vi "Logitech F310 (No Drivers).vi"(6 "error in (no error)":errorcluster, 7 "Deadzone":dbl=0.05, 8 "refnum name":string) -> (0 "Buttons":T2, 1 "D-Pad Buttons":T1, 2 "D-Pad":cluster{"X":dbl, "Y":dbl}, 3 "Right Stick":cluster{"X":dbl, "Y":dbl}, 4 "error out":errorcluster, 5 "Left Stick":cluster{"X":dbl, "Y":dbl})   [LabVIEW 2012]
uses:
  <vilib>/Rock Robotics/WPI/Joystick/WPI_JoystickGetSetRefNum.vi
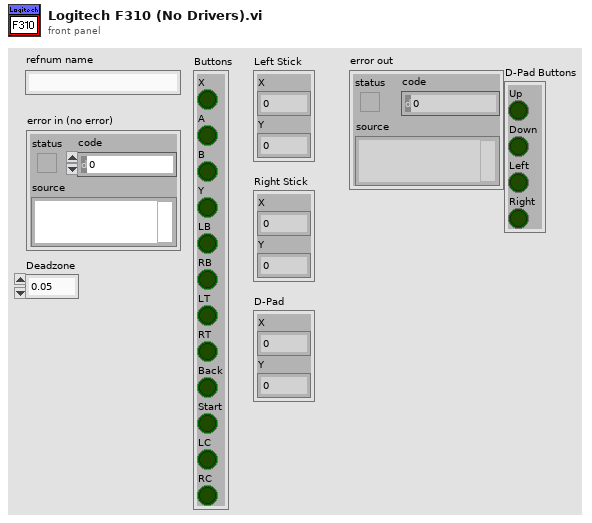
[diagram p1: front panel]
types:
  T1 = cluster{"Up":bool, "Down":bool, "Left":bool, "Right":bool}
  T2 = cluster{"X":bool, "A":bool, "B":bool, "Y":bool, "LB":bool, "RB":bool, "LT":bool, "RT":bool, "Back":bool, "Start":bool, "LC":bool, "RC":bool}
  T3 = typedef "WPI_JoystickDevRef.ctl" = cluster{"Device":T4}
  T4 = typedef "WPI_JoystickDeviceEnum.ctl" = enum16{"USB 1", "USB 2", "USB 3", "USB 4", "Kinect 1", "Kinect 2"}
  T5 = typedef "WPI_JoystickButtonState.ctl" = cluster{"Button 1":bool, "Button 2":bool, "Button 3":bool, "Button 4":bool, "Button 5":bool, "Button 6":bool, "Button 7":bool, "Button 8":bool, "Button 9":bool, "Button 10":bool, "Button 11":bool, "Button 12":bool}
  T6 = cluster{"axis 1 (x)":dbl, "axis 2 (y)":dbl, "axis 3 (throttle)":dbl, "axis 4":dbl, "axis 5":dbl, "axis 6":dbl}
  T7 = cluster{"Array(out)[0]":dbl, "Array(out)[1]":dbl, "Array(out)[2]":dbl, "Array(out)[3]":dbl, "Array(out)[4]":dbl, "Array(out)[5]":dbl}
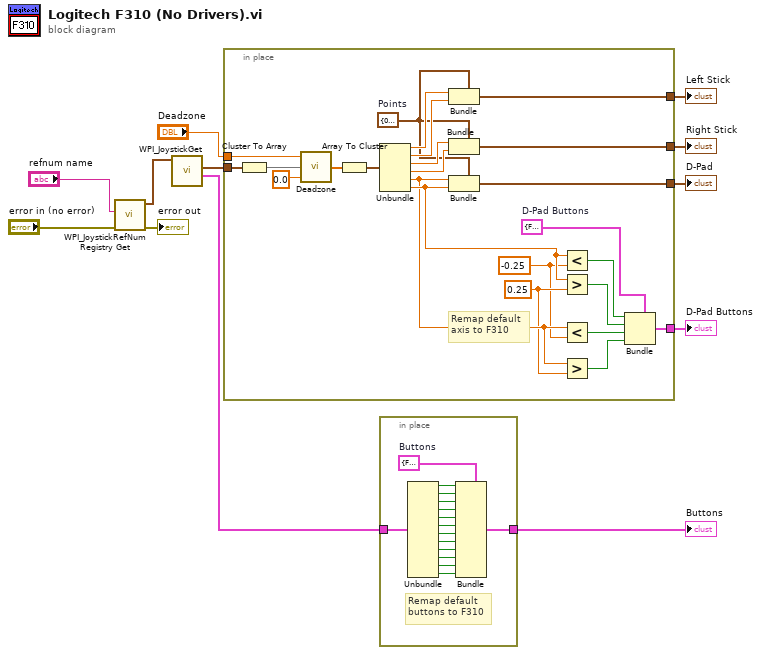
[diagram p0: block diagram]
diagram:
  n1 = call <vilib>:"WPI_JoystickRefNum Registry Get.vi"("error in (no error)"="error in (no error)", "refnum name"="refnum name") -> ("error out"=→"error out":errorcluster, "JoystickDevRef"=w12:T3)  [unwired: 8 in]
  n2 = call <vilib>:"WPI_JoystickGet.vi"("JoystickDevRef"=w12) -> ("Buttons"=w10:T5, "Axes"=w11:T6)  [unwired: 4 in, 1 out]
  n3 = in-place {
    in-place-border: w11 -> [w16]
    in-place-border: [w32] -> w6
    in-place-border: [w31] -> w5
    in-place-border: [w29] -> w4
    in-place-border: [w23] -> w2
    in-place-border: "Deadzone" -> [w13]
    w24 = -0.25 ("y")
    w25 = 0.25 ("y")
    w28 = T1 {"Up"=FALSE, "Down"=FALSE, "Left"=FALSE, "Right"=FALSE}  # D-Pad Buttons
    w30 = cluster{"X":dbl, "Y":dbl} {"X"=0.0, "Y"=0.0}  # Points
    # "Remap default\naxis to F310"
    n4 = Cluster To Array(cluster=w16) -> (array=w18:dbl[])
    n5 = call "Deadzone.vi"("Default"=0.0, "Array(in)"=w18, "Deadzone"=w13) -> ("Array(out)"=w17:dbl[])  [unwired: 2 in]
    n6 = Array To Cluster(array=w17) -> (cluster=w15:T7)
    n7 = Unbundle(w15) -> ("Array(out)[0]"=w36:dbl, "Array(out)[1]"=w35:dbl, "Array(out)[2]"=w34:dbl, "Array(out)[3]"=w33:dbl, "Array(out)[4]"=w26:dbl, "Array(out)[5]"=w27:dbl)
    n8 = Bundle(cluster=w30, "X"=w36, "Y"=w35) -> (w32:cluster{"X":dbl, "Y":dbl})
    n9 = Bundle(cluster=w30, "X"=w34, "Y"=w33) -> (w31:cluster{"X":dbl, "Y":dbl})
    n10 = Bundle(cluster=w30, "X"=w26, "Y"=w27) -> (w29:cluster{"X":dbl, "Y":dbl})
    n11 = Less?(x=w27, y=w24) -> (x < y?=w21:bool)
    n12 = Greater?(x=w27, y=w25) -> (0:w22:bool)
    n13 = Less?(x=w26, y=w24) -> (x < y?=w19:bool)
    n14 = Greater?(x=w26, y=w25) -> (0:w20:bool)
    n15 = Bundle(cluster=w28, "Up"=w21, "Down"=w22, "Left"=w19, "Right"=w20) -> (w23:T1)
  }
  "Left Stick" <- w6
  "Right Stick" <- w5
  "D-Pad" <- w4
  "D-Pad Buttons" <- w2
  n16 = in-place {
    in-place-border: w10 -> [w51]
    in-place-border: [w37] -> w3
    w50 = T2 {"X"=FALSE, "A"=FALSE, "B"=FALSE, "Y"=FALSE, "LB"=FALSE, "RB"=FALSE, "LT"=FALSE, "RT"=FALSE, "Back"=FALSE, "Start"=FALSE, "LC"=FALSE, "RC"=FALSE}  # Buttons
    # "Remap default\nbuttons to F310"
    n17 = Unbundle(w51) -> ("Button 1"=w49:bool, "Button 2"=w48:bool, "Button 3"=w47:bool, "Button 4"=w46:bool, "Button 5"=w45:bool, "Button 6"=w44:bool, "Button 7"=w43:bool, "Button 8"=w42:bool, "Button 9"=w41:bool, "Button 10"=w40:bool, "Button 11"=w39:bool, "Button 12"=w38:bool)
    n18 = Bundle(cluster=w50, "X"=w49, "A"=w48, "B"=w47, "Y"=w46, "LB"=w45, "RB"=w44, "LT"=w43, "RT"=w42, "Back"=w41, "Start"=w40, "LC"=w39, "RC"=w38) -> (w37:T2)
  }
  "Buttons" <- w3
